vi "UHR-Fleezers Control (host) -Leonardo 04-2018 V3_greenctrl.vi"(0 "Tab Green FB":T5(tab)=enum."Trap Control (RF)") -> ()   [LabVIEW 2013] (continued)
                    n952 = call "Write to pump.vi"("string"="start", "VISA resource name"=w1530) -> ()  [unwired: 1 out]
                  }
                  frame #3 {
                    n953 = Wait (ms)(milliseconds to wait=u32 500) -> ()  [unwired: 1 out]
                  }
                  frame #4 {
                    n954 = call "Write to pump.vi"("string"="start", "VISA resource name"=w1534) -> ()  [unwired: 1 out]
                  }
                }
              }
            }
          }
          frame Enabled {
            n955 = call "hamilton_controller.vi"("Open?"=w1536, "valve"=enum16{"A", "B", "C", "D", "ALL"}."A", "action"=T21."MOVE VALVE") -> ()  [unwired: 8 in, 1 out]
          }
        }
      }
      event "Inject Valve B": Value Change {
        n956 = event-data() -> ()  [unwired: 7 out]
        n957 = disable-structure shown="Enabled" {
          disable-tunnel: "Inject Valve B" -> [w1540 w1560]
          frame Disabled {
            n958 = local read "Pump write delay (ms)"() -> (w1542:dbl)
            n959 = flat-sequence {
              tunnel: w1541 -> [w1555]
              tunnel: w1542 -> [w1551]
              tunnel: w1540 -> [_]
              tunnel: w1542 -> [w1557]
              tunnel: w1541 -> [w1558]
              frame #0 {
                n960 = local read "All Pump Parameters"() -> (w1550:T6)
                n961 = Multiply(x=60.0, y="Flush Center Ch Rate (ul/m)") -> (x*y=w1547:dbl)
                n962 = Unbundle By Name(w1550) -> ("Pump 2"=w1556:T33)
                n963 = call "Set pump parameters.vi"("Pump write delay (ms)"=w1551, "Volume (uL)"="Flush Center Ch Volume (uL)", "Rate (uL/h)"=w1547, "Units"=3.0, "Pump #"=2.0, "Pump Parameters In"=w1556, "VISA resource name"=w1555) -> ("Pump Parameters Out"=w1549:T33)  [unwired: 3 in]
                n964 = Bundle By Name(cluster=w1550, "Pump 2"=w1549) -> (w1548:T6)
                n965 = local write "All Pump Parameters"(w1548) -> ()
                n966 = Add(x="Flush Center Ch Volume (uL)", y="Total Volume\nFlushed (uL)") -> (x+y=w1544:dbl)
                n967 = local write "Total Volume\nFlushed (uL)"(w1544) -> ()
              }
              frame #1 {
                n968 = Wait (ms)(milliseconds to wait=w1557) -> ()  [unwired: 1 out]
              }
              frame #2 {
                n969 = call "Write to pump.vi"("string"="start", "VISA resource name"=w1558) -> ()  [unwired: 1 out]
              }
            }
            n970 = local read "Chemyx Syringe Pump Serial Port"() -> (w1541:refnum<visa-resource-name>)
          }
          frame Enabled {
            n971 = call "hamilton_controller.vi"("Open?"=w1560, "valve"=enum16{"A", "B", "C", "D", "ALL"}."B", "action"=T21."MOVE VALVE") -> ()  [unwired: 8 in, 1 out]
          }
        }
      }
      event "Inject Bottom": Value Change {
        n972 = event-data() -> ()  [unwired: 7 out]
        n973 = call "hamilton_controller.vi"("Open?"="Inject Bottom", "valve"=enum16{"A", "B", "C", "D", "ALL"}."C", "action"=T21."MOVE VALVE") -> ()  [unwired: 8 in, 1 out]
      }
      event "Shunt:": Value Change {
        n974 = event-data() -> ()  [unwired: 7 out]
        n975 = call "hamilton_controller.vi"("Open?"="Shunt:", "valve"=enum16{"A", "B", "C", "D", "ALL"}."D", "action"=T21."MOVE VALVE") -> ()  [unwired: 8 in, 1 out]
      }
      event "Flip Green Filter": Value Change {
        n976 = event-data() -> ()  [unwired: 7 out]
        n977 = local write "Flip Green Filter"("Flip Green Filter") -> ()
        n978 = flat-sequence {
          tunnel: w1576 -> [w1581]
          tunnel: w1575 -> [w1580]
          tunnel: [w1578] -> w1573
          tunnel: [w1577] -> w1572
          tunnel: [w1583] -> w1571
          tunnel: w1573 -> [w1583]
          tunnel: [w1582] -> w1570
          tunnel: w1572 -> [w1582]
          tunnel: w1571 -> [w1587]
          tunnel: w1570 -> [w1586]
          tunnel: [w1585] -> w1574
          frame #0 {
            n979 = xnode "Read/Write Control"("FPGA VI Reference In"=w1581, "error in"=w1580, "Green Filter Flipper"=TRUE) -> ("FPGA VI Reference Out"=w1578:T20, "error out"=w1577:errorcluster)
          }
          frame #1 {
            n980 = Wait (ms)(milliseconds to wait=u32 100) -> ()  [unwired: 1 out]
          }
          frame #2 {
            n981 = xnode "Read/Write Control"("FPGA VI Reference In"=w1587, "error in"=w1586, "Green Filter Flipper"=FALSE) -> ("error out"=w1585:errorcluster)  [unwired: 1 out]
          }
        }
      }
      event "Pump 1 contents", "Pump 3 contents": Value Change {
        n982 = event-data() -> ()  [unwired: 7 out]
        n983 = local read "Pump 1 contents"() -> (→"Pump 1 cont disp":string)
        n984 = local read "Pump 3 contents"() -> (→"Pump 3 cont disp":string)
      }
      event "Reset Trap Pos. FB": Value Change {
        n985 = event-data() -> ()  [unwired: 7 out]
        n986 = xnode "Read/Write Control"("FPGA VI Reference In"=w1593, "error in"=w1592, "Trap Pos. FB Reset"="Reset Trap Pos. FB") -> ()  [unwired: 2 out]
      }
      event "Trap Pos. FB ON": Value Change {
        n987 = event-data() -> ()  [unwired: 7 out]
        n988 = xnode "Read/Write Control"("FPGA VI Reference In"=w1608, "error in"=w1607) -> ("FPGA VI Reference Out"=w1605:T20, "BD1 Frequency Out 1"=w1602:u64)  [unwired: 1 out]
        n989 = To Double Precision Float(number=w1602) -> (double precision float=w1601:dbl)
        n990 = Multiply(x=49125000.0, y=6.0) -> (x*y=w1600:dbl)
        n991 = Multiply(x=w1601, y=w1600) -> (x*y=w1598:dbl)
        n992 = Scale By Power Of 2(n=-48, x=w1598) -> (x*2^n=w1597:dbl)
        n993 = Divide(x=w1597, y=1000000.0) -> (x/y=w1594:dbl)
        n994 = flat-sequence {
          tunnel: [w1611] -> w1606
          tunnel: w1605 -> [w1612]
          tunnel: w1602 -> [w1610]
          tunnel: "Trap Pos. FB ON" -> [w1609]
          tunnel: "Trap Pos. FB ON" -> [w1618]
          tunnel: w1606 -> [w1617]
          tunnel: "Trap Pos. FB ON" -> [w1620]
          tunnel: w1594 -> [w1619]
          frame #0 {
            n995 = case shown="False" w1609 {
              tunnel: w1612 -> [w1615 w1616]
              tunnel: [w1614 w1616] -> w1611
              tunnel: w1610 -> [w1613 _]
              frame False {
                n996 = xnode "Read/Write Control"("FPGA VI Reference In"=w1615, "BD 1 Frequency 1"=w1613) -> ("FPGA VI Reference Out"=w1614:T20)  [unwired: 1 in, 1 out]
              }
              frame True {
              }
            }
          }
          frame #1 {
            n997 = xnode "Read/Write Control"("FPGA VI Reference In"=w1617, "Force feedback"=w1618) -> ()  [unwired: 1 in, 2 out]
          }
          frame #2 {
            n998 = case shown="False" w1620 {
              tunnel: w1619 -> [w1623 _]
              frame False {
                n999 = local read "T2 for asymmetric\n(MHz)"() -> (w1621:dbl)
                n1000 = Subtract(x=w1621, y=w1623) -> (x-y=w1622:dbl)
                n1001 = property on="Trap Delta (MHz)" class="DigNum (strict)"("Val(Sgnl)"=w1622) -> ()  [unwired: 2 in, 2 out]
              }
              frame True {
              }
            }
          }
        }
      }
      event "Diff. FB.", "Trap Pos. FB Gains", "Trap Pos. FB Mult Factor", "Trap Pos. FB Offset Factor", "Trap Pos FB Negate Action", "Trap Pos FB Monitor\nT1 or T2", "Negate Diff?": Value Change {
        n1002 = event-data() -> ()  [unwired: 7 out]
        n1003 = xnode "Read/Write Control"("FPGA VI Reference In"=w1634, "error in"=w1633, "Trap pos. FB Range"="Trap Pos. FB Range", "Trap Pos. FB Gains"="Trap Pos. FB Gains", "Trap Pos. FB Mult Factor"="Trap Pos. FB Mult Factor", "Trap Pos. FB Offset Factor"="Trap Pos. FB Offset Factor", "Trap Pos FB Negate Action"="Trap Pos FB Negate Action", "Trap Pos FB Monitor T1 or T2"="Trap Pos FB Monitor\nT1 or T2", "AI1 X Scale"="Trap Pos. AI1 X Pre-scale", "Negate Diff?"="Negate Diff?", "Diff FB Measurement?"="Diff. FB.") -> ()  [unwired: 2 out]
      }
      event "Trap Pos FB SP": Value Change {
        n1004 = event-data() -> ()  [unwired: 7 out]
        n1005 = xnode "Read/Write Control"("FPGA VI Reference In"=w1637, "error in"=w1636, "Trap Pos. FB SP"="Trap Pos FB SP") -> ()  [unwired: 2 out]
        n1006 = disable-structure shown="Disabled" {
          frame Disabled {
            n1007 = local read "Trap X AI1 (DMA)"() -> (w1658:T13)
            n1008 = local read "Trap X (AI1)"() -> (w1659:T1)
            n1009 = local read "Setpoint offset\nCorrection values"() -> (w1652:dbl[])
            n1010 = local read "Trap Delta (MHz)"() -> (w1656:dbl)
            n1011 = local read "B factor"() -> (w1643:dbl)
            n1012 = Unbundle(w1659) -> ("Trap 1"=w1657:fxp<+/-,16,1>, "Trap 2"=w1646:fxp<+/-,16,1>)
            n1013 = Unbundle(w1658) -> ("Set 1"=w1642:fxp<+/-,16,1>, "Set 2"=w1641:fxp<+/-,16,1>)
            n1014 = Negate(x=w1646) -> (-x=w1639:fxp<+/-,17,2>)
            n1015 = Negate(x=w1657) -> (-x=w1640:fxp<+/-,17,2>)
            n1016 = Divide(x=w1656, y=0.1) -> (x/y=w1654:dbl)
            n1017 = Multiply(x=w1641, y=w1643) -> (x*y=w1644:dbl)
            n1018 = Subtract(x=w1642, y=w1644) -> (x-y=w1649:dbl)
            n1019 = To Long Integer(number=w1654) -> (32bit integer=w1653:i32)
            n1020 = Index Array(array=w1652, index=w1653) -> (element=w1648:dbl)
            n1021 = Multiply(x=w1643, y=w1639) -> (x*y=w1645:dbl)
            n1022 = Subtract(x=w1640, y=w1645) -> (x-y=w1651:dbl)
            n1023 = Add(x=w1651, y=w1648) -> (x+y=→"ideal setpoint fpga":dbl)
            n1024 = Add(x=w1649, y=w1648) -> (x+y=→"ideal setpoint avgd":dbl)
          }
          frame Enabled {
          }
        }
        n1025 = disable-structure shown="Enabled" {
          frame Enabled {
          }
          frame Disabled {
            n1026 = local write "B factor"(1.0 ("B factor")) -> ()
          }
        }
      }
      event "Simulate stepping": Value Change {
        n1027 = event-data() -> ()  [unwired: 7 out]
        n1028 = flat-sequence {
          tunnel: w1661 -> [w1664]
          tunnel: [w1663] -> _
          tunnel: w1660 -> [w1662]
          frame #0 {
            n1029 = while {
              tunnel: w1664 -> [w1692]
              tunnel: [w1691] -> w1663 mode=indexing
              tunnel: w1662 -> [w1690]
              i -> [w1676]
              stop <- w1673 stop-if-true
              w1666 = 1000.0
              n1030 = Divide(x="Backtrack probability", y=100) -> (x/y=w1700:dbl)
              n1031 = Random Number (0-1)() -> (number: 0 to 1=w1701:dbl)
              n1032 = Greater?(x=w1701, y=w1700) -> (0:w1699:bool)
              n1033 = Select(t=1, s=w1699, f=-1) -> (s? t:f=w1696:i32)
              n1034 = local read "BD 1 Frequency 2 (MHz)"() -> (w1671:dbl)
              n1035 = Multiply(x=w1696, y="Step size (nm)") -> (x*y=w1694:dbl)
              "Step taken" <- w1694
              n1036 = Divide(x=w1694, y=168.33) -> (x/y=w1669:dbl)
              n1037 = local read "BD 1 Frequency 1 (MHz)"() -> (w1670:dbl)
              n1038 = local read "X RF Frequency Limits (MHz)"() -> (w1689:T16)
              n1039 = local read "Y RF Frequency Limits (MHz)"() -> (w1688:T16)
              n1040 = Subtract(x=w1670, y=w1669) -> (x-y=w1668:dbl)
              n1041 = local write "BD 1 Frequency 1 (MHz)"(w1668) -> ()
              n1042 = local read "BD 2 Frequency 1 (MHz)"() -> (w1686:dbl)
              n1043 = local read "BD 2 Frequency 2 (MHz)"() -> (w1687:dbl)
              n1044 = call "set RF board frequency - interlace.vi"("Board 2 Frequency Limits"=w1688, "Board 1 Frequency Limits"=w1689, "error in"=w1692, "FPGA VI Reference In"=w1690, "Board 2 Frequency 2 (MHz)"=w1687, "Board 2 Frequency 1 (MHz)"=w1686, "Board 1 Frequency 2 (MHz)"=w1671, "Board 1 Frequency 1  (MHz)"=w1668) -> ("error out"=w1691:errorcluster)  [unwired: 2 in, 1 out]
              n1045 = Subtract(x=w1671, y=w1668) -> (x-y=w1685:dbl)
              n1046 = Subtract(x=w1687, y=w1686) -> (x-y=w1684:dbl)
              n1047 = Square(x=w1684) -> (x^2=w1682:dbl)
              n1048 = Square(x=w1685) -> (x^2=w1683:dbl)
              n1049 = Add(x=w1683, y=w1682) -> (x+y=w1681:dbl)
              n1050 = Square Root(x=w1681) -> (sqrt(x)=w1672:dbl)
              n1051 = local write "Trap Delta (MHz)"(w1672) -> ()
              n1052 = property on="Initial delta (MHz)" class="DigNum (strict)"("Val(Sgnl)"=w1672) -> ()  [unwired: 2 in, 2 out]
              n1053 = Multiply(x="Mean dwell time (s)", y=w1666) -> (x*y=w1678:dbl)
              n1054 = case shown="\"Gamma2\"" "Distribution" {
                tunnel: w1678 -> [w1705 w1709 w1712]
                tunnel: [w1705 w1706 w1713] -> w1667
                frame "uniform", Default {
                }
                frame "Exponential" {
                  n1055 = call-poly <vilib>:"Continuous Random.vi"("b"=w1709, "samples"=1) -> ("exp random data"=w1707:dbl[])  [unwired: 8 in, 1 out]
                  n1056 = Index Array(array=w1707) -> (element=w1706:dbl)  [unwired: 1 in]
                }
                frame "Gamma2" {
                  w1710 = 2.0
                  # "Note: the shape and scale\nparameters of the gamma\nare inverted because LabView..."
                  n1057 = Divide(x=w1712, y=w1710) -> (x/y=w1711:dbl)
                  n1058 = call-poly <vilib>:"Continuous Random.vi"("c"=w1711, "b"=w1710, "samples"=1) -> ("gamma random numbers"=w1714:dbl[])  [unwired: 7 in, 1 out]
                  n1059 = Index Array(array=w1714) -> (element=w1713:dbl)  [unwired: 1 in]
                }
              }
              n1060 = Divide(x=w1667, y=w1666) -> (x/y=→"Step duration":dbl)
              n1061 = To Unsigned Long Integer(number=w1667) -> (unsigned 32bit integer=w1679:u32)
              n1062 = Add(x=w1676, y=1) -> (x+y=w1675:i32)
              n1063 = Wait (ms)(milliseconds to wait=w1679) -> ()  [unwired: 1 out]
              n1064 = Equal?(x=w1675, y="Number of steps") -> (x = y?=w1673:bool)
            }
          }
          frame #1 {
            n1065 = local write "Simulate stepping"(FALSE) -> ()
          }
        }
      }
      event "Set SP to Reading": Value Change {
        n1066 = event-data() -> ()  [unwired: 7 out]
        n1067 = local read "Trap Pos FB Monitor\nT1 or T2"() -> (w1724:bool)
        n1068 = local read "Trap X AI1 (DMA)"() -> (w1727:T13)
        n1069 = local read "Trap X (AI1)"() -> (w1730:T1)
        n1070 = Unbundle By Name(w1730) -> ("Trap 1"=w1729:fxp<+/-,16,1>, "Trap 2"=w1728:fxp<+/-,16,1>)
        n1071 = Unbundle By Name(w1727) -> ("Set 1"=w1726:fxp<+/-,16,1>, "Set 2"=w1725:fxp<+/-,16,1>)
        n1072 = Select(t=w1729, s=w1724, f=w1728) -> (s? t:f=w1723:fxp<+/-,16,1>)
        n1073 = Select(t=w1726, s=w1724, f=w1725) -> (s? t:f=w1722:fxp<+/-,16,1>)
        n1074 = Not(x="Set SP Using...") -> (.not. x?=w1717:bool)
        n1075 = Select(t=w1723, s=w1717, f=w1722) -> (s? t:f=w1718:fxp<+/-,16,1>)
        n1076 = xnode "Read/Write Control"("FPGA VI Reference In"=w1720, "error in"=w1719, "Trap Pos. FB SP"=w1718) -> ()  [unwired: 2 out]
        n1077 = local write "Trap Pos FB SP"(w1718) -> ()
      }
      event "Trap Pos. FB Out Scale 2^n": Value Change {
        n1078 = event-data() -> ()  [unwired: 7 out]
        n1079 = Scale By Power Of 2(n="Trap Pos. FB Out Scale 2^n", x=ext 1.0) -> (x*2^n=w1732:ext)
        n1080 = property on="Trap Pos. FB Mult Factor" class="DigNum (strict)"("Val(Sgnl)"=w1732) -> ()  [unwired: 2 in, 2 out]
      }
      event "Trap Pos FB Int Count": Value Change {
        n1081 = event-data() -> ()  [unwired: 7 out]
        n1082 = xnode "Read/Write Control"("FPGA VI Reference In"=w1737, "error in"=w1736, "Trap Pos FB Int Count"="Trap Pos FB Int Count") -> ()  [unwired: 2 out]
      }
      event "Target Force (pN)", "Setpoint offset\nCorrection values", "Raster target force (pN)": Value Change {
        w1746 = 2.0
        n1083 = event-data() -> ()  [unwired: 7 out]
        n1084 = disable-structure "Removed B Factor to improve position feedback - Alex 081418 1of3" shown="Enabled" {
          disable-tunnel: [w1776 fxp<+/-,32,16> 1.0 ("B factor")] -> w1738
          frame Disabled {
            n1085 = local read "B factor"() -> (w1777:dbl)
            n1086 = To Fixed-Point(number=w1777) -> (fixed-point=w1776:fxp<+/-,16,16>)  [unwired: 1 in]
          }
          frame Enabled {
          }
        }
        n1087 = xnode "Read/Write Control"("FPGA VI Reference In"=w1740, "B factor"=w1738) -> ("BD1 Frequency Out 1"=w1767:u64)  [unwired: 1 in, 2 out]
        n1088 = local read "BD 1 Frequency 2 (MHz)"() -> (w1766:dbl)
        n1089 = local read "Target Force (pN)"() -> (w1752:dbl)
        n1090 = To Double Precision Float(number=w1767) -> (double precision float=w1773:dbl)
        n1091 = Multiply(x=49125000.0, y=6.0) -> (x*y=w1772:dbl)
        n1092 = Multiply(x=w1773, y=w1772) -> (x*y=w1770:dbl)
        n1093 = Scale By Power Of 2(n=-48, x=w1770) -> (x*2^n=w1769:dbl)
        n1094 = Divide(x=w1769, y=1000000.0) -> (x/y=w1765:dbl)
        n1095 = Subtract(x=w1766, y=w1765) -> (x-y=w1764:dbl)
        n1096 = local read "T1 kappa_x (pN/nm)"() -> (w1753:dbl)
        n1097 = local read "T1 alpha_x (nm/V)"() -> (w1754:dbl)
        n1098 = local read "Negate offset difference"() -> (w1755:bool)
        n1099 = local read "Offset file step size"() -> (w1763:dbl)
        n1100 = Multiply(x="Raster target force (pN)", y=w1746) -> (x*y=w1745:dbl)
        n1101 = Multiply(x=w1752, y=w1746) -> (x*y=w1751:dbl)
        n1102 = local read "Setpoint offset\nCorrection values"() -> (w1760:dbl[])
        n1103 = Divide(x=w1764, y=w1763) -> (x/y=w1762:dbl)
        n1104 = Select(t=-1, s=w1755, f=1) -> (s? t:f=w1756:i32)
        n1105 = To Long Integer(number=w1762) -> (32bit integer=w1761:i32)
        n1106 = Multiply(x=w1754, y=w1753) -> (x*y=w1744:dbl)
        n1107 = Divide(x=w1751, y=w1744) -> (x/y=w1750:dbl)
        n1108 = Index Array(array=w1760, index=w1761) -> (element=w1759:dbl)
        n1109 = Divide(x=w1745, y=w1744) -> (x/y=w1743:dbl)
        n1110 = Multiply(x=w1756, y=w1759) -> (x*y=w1742:dbl)
        n1111 = Add(x=w1750, y=w1742) -> (x+y=w1749:dbl)
        n1112 = Add(x=w1743, y=w1742) -> (x+y=w1741:dbl)
        n1113 = To Fixed-Point(number=w1741) -> (fixed-point=w1739:fxp<+/-,16,1>)  [unwired: 1 in]
        n1114 = To Fixed-Point(number=w1749) -> (fixed-point=w1748:fxp<+/-,16,1>)  [unwired: 1 in]
        n1115 = property on="Trap Pos FB SP" class="DigNum (strict)"("Val(Sgnl)"=w1748) -> ()  [unwired: 2 in, 2 out]
        n1116 = xnode "Read/Write Control"("FPGA VI Reference In"=w1740, "Raster setpoint"=w1739) -> ()  [unwired: 1 in, 2 out]
      }
      event "Read setpoint correction\nfile": Value Change {
        n1117 = event-data() -> ()  [unwired: 7 out]
        n1118 = local write "Read setpoint correction\nfile"(FALSE) -> ()
        n1119 = Open/Create/Replace File(file path (use dialog)="Setpoint correction\noffset file", operation (0:open)=T24."open", access (0:read/write)=enum16{"read/write", "read-only", "write-only"}."read-only") -> (refnum out=w1804:refnum<file>)  [unwired: 1 in, 4 out]
        n1120 = Deny Access(7:w1804) -> (3:w1802:refnum<file>)  [unwired: 1 in, 2 out]
        n1121 = Read from Binary File(5:0.0, 9:T30."big-endian, network order" ("byte order (0:big-endian, network order)"), 10:-1 ("count (1)"), 11:w1802) -> (2:w1795:dbl[], 3:w1801:refnum<file>)  [unwired: 1 in, 3 out]
        n1122 = Close File(refnum=w1801) -> ()  [unwired: 1 in, 2 out]
        n1123 = Index Array(array=w1795, index=0) -> (element=w1791:dbl)
        n1124 = local write "Offset file step size"(w1791) -> ()
        n1125 = Array Subset(array=w1795, index=3) -> (w1794:dbl[])  [unwired: 1 in]
        n1126 = local read "T1 kappa_x (pN/nm)"() -> (w1789:dbl)
        n1127 = local read "T1 alpha_x (nm/V)"() -> (w1790:dbl)
        n1128 = local read "T2 alpha_x (nm/V)"() -> (w1788:dbl)
        n1129 = local read "T2 kappa_x (pN/nm)"() -> (w1787:dbl)
        n1130 = Decimate 1D Array(w1794) -> (w1783:dbl[], w1784:dbl[])  [unwired: 1 out]
        n1131 = local read "Offset Values"() -> (w1793:T14)
        n1132 = Multiply(x=w1790, y=w1789) -> (x*y=w1785:dbl)
        n1133 = Multiply(x=w1788, y=w1787) -> (x*y=w1786:dbl)
        n1134 = Bundle By Name(cluster=w1793, "Trap 1X offset"=w1783, "Trap 2X offset"=w1784) -> (w1792:T14)
        n1135 = Divide(x=w1786, y=w1785) -> (x/y=w1780:dbl)
        n1136 = disable-structure "Removed B Factor to better position FB - Alex 081418 3of3" shown="Enabled" {
          disable-tunnel: w1780 -> [w1808 _]
          disable-tunnel: [w1808 1.0] -> w1779
          frame Disabled {
          }
          frame Enabled {
          }
        }
        n1137 = Multiply(x=w1784, y=w1779) -> (x*y=w1782:dbl[])
        n1138 = local write "Offset Values"(w1792) -> ()
        n1139 = Subtract(x=w1783, y=w1782) -> (x-y=w1781:dbl[])
        n1140 = property on="B factor" class="DigNum (strict)"("Val(Sgnl)"=w1779) -> ()  [unwired: 2 in, 2 out]
        n1141 = property on="Setpoint offset\nCorrection values" class="Arr (strict)"("Val(Sgnl)"=w1781) -> ()  [unwired: 2 in, 2 out]
      }
      event "MCL Tracking": Value Change {
        n1142 = event-data() -> ()  [unwired: 7 out]
        n1143 = case shown="True" "MCL Tracking" {
          frame False {
            n1144 = local read "Current MCL (V)"() -> (w1811:dbl)
            n1145 = local write "AO2"(w1811) -> ()
          }
          frame True {
            n1146 = local read "BD 1 Frequency 1 (MHz)"() -> (→"Zero T1 position":dbl)
            n1147 = local read "AO2"() -> (→"Zero MCL x position":dbl)
          }
        }
      }
      event "Scale intensities": Value Change {
        n1148 = event-data() -> ()  [unwired: 7 out]
        n1149 = local read "Trap Intensity\nSetpoints (V)"() -> (w1817:cluster{"Set 1":dbl, "Set 2":dbl})
        n1150 = local read "T1 kappa_x (pN/nm)"() -> (w1823:dbl)
        n1151 = local read "T2 kappa_x (pN/nm)"() -> (w1822:dbl)
        n1152 = Unbundle By Name(w1817) -> ("Set 1"=w1819:dbl, "Set 2"=w1818:dbl)
        n1153 = case shown="True" "Scale intensities" {
          tunnel: "Scale factor" -> [w1833 w1845]
          tunnel: "Scale factor" -> [w1828 w1838]
          tunnel: w1823 -> [w1835 w1844]
          tunnel: w1822 -> [w1834 w1843]
          tunnel: [w1831 w1842] -> w1821
          tunnel: [w1832 w1841] -> w1820
          tunnel: w1819 -> [w1830 w1840]
          tunnel: w1818 -> [w1829 w1839]
          tunnel: [w1827 w1837] -> w1816
          tunnel: [w1826 w1836] -> w1815
          frame False {
            n1154 = Divide(x=w1835, y=w1828) -> (x/y=w1831:dbl)
            n1155 = Divide(x=w1834, y=w1833) -> (x/y=w1832:dbl)
            n1156 = Divide(x=w1830, y=w1828) -> (x/y=w1827:dbl)
            n1157 = Divide(x=w1829, y=w1828) -> (x/y=w1826:dbl)
          }
          frame True {
            n1158 = Multiply(x=w1840, y=w1838) -> (x*y=w1837:dbl)
            n1159 = Multiply(x=w1839, y=w1838) -> (x*y=w1836:dbl)
            n1160 = Multiply(x=w1844, y=w1838) -> (x*y=w1842:dbl)
            n1161 = Multiply(x=w1845, y=w1843) -> (x*y=w1841:dbl)
          }
        }
        n1162 = local write "T2 kappa_x (pN/nm)"(w1820) -> ()
        n1163 = local write "T1 kappa_x (pN/nm)"(w1821) -> ()
        n1164 = Bundle By Name(cluster=w1817, "Set 1"=w1816, "Set 2"=w1815) -> (w1814:cluster{"Set 1":dbl, "Set 2":dbl})
        n1165 = property on="Trap Intensity\nSetpoints (V)" class="Clust (strict)"("Val(Sgnl)"=w1814) -> ()  [unwired: 2 in, 2 out]
      }
    }
    "error out 2" <- w772
    n1166 = node-c288() -> ()  [unwired: 1 in, 1 out]
  }
  n1167 = node-c288() -> (w103:T25)  [unwired: 4 in]
  n1168 = timed-loop "Run Scripts, including: stage motion" {
    timing: w103 -> [_]
    timing-out: [_] -> w102
    tunnel: w61 -> [_]
    stop <- w1847 stop-if-true
    n1169 = node-c288() -> ()  [unwired: 1 in, 1 out]
    n1170 = event shown="[0] \"Move Cap. 1 (DNA Top)\": Value Change" {
      selector: _ -> [_ _ _ _ _ _ _ _ _ _ _ _]
      dyn-events: _ -> [_ _ _ _ _ _ _ _ _ _ _ _]
      timeout: 50 -> [_ _ _ _ _ _ _ _ _ _ _ _]
      tunnel: ["Move Cap. 1 (DNA Top)" _ "Cal/Data Acq. Spot" "Dump Beads" "Dip for Protein" _ "Got ADig bead" "Got DNA bead" "Take Stepping Data" _ "Take Detection Laser\nImage" _] -> _
      tunnel: [_ _ _ _ _ _ _ _ _ _ _ w2057] -> w1847
      event "Move Cap. 1 (DNA Top)": Value Change {
        n1171 = event-data() -> ()  [unwired: 1 in, 5 out]
        n1172 = local write "Move Cap. 1 (DNA Top)"(FALSE ("Move Cap. 1 (DNA Right)")) -> ()
        n1173 = flat-sequence {
          tunnel: "Cap 1 Samp Flow ON" -> [w1853]
          frame #0 {
            n1174 = local write "Stage Moving"(FALSE ("Stage Moving")) -> ()
            n1175 = case "stop flow" shown="True" w1853 {
              frame False {
              }
              frame True {
                n1176 = call "hamilton_controller.vi"("Open?"=FALSE, "valve"=enum16{"A", "B", "C", "D", "ALL"}."C", "action"=T21."MOVE VALVE") -> ()  [unwired: 8 in, 1 out]
              }
            }
            n1177 = case shown="True" TRUE {
              tunnel: "Cap 1 T ON" -> [w1862 w1863]
              frame False {
                n1178 = property on="Trap 1 (ON/OFF)" class="Bool (strict)"("Val(Sgnl)"=w1862) -> ()  [unwired: 2 in, 2 out]
              }
              frame True {
                n1179 = property on="Trap 2 (ON/OFF)" class="Bool (strict)"("Val(Sgnl)"=w1863) -> ()  [unwired: 2 in, 2 out]
              }
            }
            n1180 = call <vilib>:"Beep.vi"() -> ()  [unwired: 3 in, 9 out]
            n1181 = case shown="True" "Cap 1 Flow ON" {
              frame False {
              }
              frame True {
                n1182 = property on="Main:" class="Bool (strict)"("Val(Sgnl)"=TRUE ("Value (Signaling)")) -> ()  [unwired: 2 in, 2 out]
              }
            }
          }
        }
      }
      event Timeout {
        n1183 = event-data() -> ()  [unwired: 1 in, 2 out]
      }
      event "Cal/Data Acq. Spot": Value Change {
        # "wait for calibration file\nto be written"
        # "signal save cal true\nthis tells the data \nacquisition loop to\nstart sending the data\nto a calibration file"
        # "separate traps to\nthe desired trap delta"
        # "move stage to data acquisition spot"
        # "CHANGE FISH FOR TETHER BACK\nTO TRUE VALUE HERE."
        n1184 = event-data() -> ()  [unwired: 1 in, 5 out]
        n1185 = flat-sequence {
          tunnel: ["Cal @ (MHz)"] -> w1864
          tunnel: w1864 -> [w1876]
          tunnel: w1864 -> [w1897]
          frame #0 {
            n1186 = property on="Trap Delta (MHz)" class="DigNum (strict)"("Val(Sgnl)"="Cal @ (MHz)") -> ()  [unwired: 2 in, 2 out]
            n1187 = call <vilib>:"Beep.vi"() -> ()  [unwired: 3 in, 9 out]
          }
          frame #1 {
            n1188 = local read "Scale intensities"() -> (w1868:bool)
            n1189 = case shown="True" w1868 {
              frame False {
              }
              frame True {
                n1190 = property on="Scale intensities" class="Bool (strict)"("Val(Sgnl)"=FALSE ("Value (Signaling)")) -> ()  [unwired: 2 in, 2 out]
              }
            }
          }
          frame #2 {
            n1191 = Wait (ms)(milliseconds to wait=u32 500) -> ()  [unwired: 1 out]
          }
          frame #3 {
            n1192 = property on="Save Calibration" class="Bool (strict)"("Val(Sgnl)"=TRUE ("Value (Signaling)")) -> ()  [unwired: 2 in, 2 out]
          }
          frame #4 {
            n1193 = Wait (ms)(milliseconds to wait=u32 4000) -> ()  [unwired: 1 out]
          }
          frame #5 {
            n1194 = while {
              stop <- w1873 stop-if-true
              n1195 = local read "Saving..."() -> (w1874:bool)
              n1196 = Wait (ms)(milliseconds to wait=u32 100) -> ()  [unwired: 1 out]
              n1197 = Not(x=w1874) -> (.not. x?=w1873:bool)
            }
          }
          frame #6 {
            n1198 = case shown="True" "W/ Offset 1" {
              tunnel: w1876 -> [_ w1878]
              frame False {
              }
              frame True {
                n1199 = stacked-sequence {
                  tunnel: w1878 -> [_ _ _ _ _ _ _ w1895]
                  frame #0 {
                    n1200 = Replace Array Subset(array=u32[] [0] ("Index Values"), new element="Offset 1 Set", index=0) -> (w1879:u32[])
                    n1201 = property on="Saved AOD Raster Scan Parameter Sets" class="Arr (strict)"("Index Values"=w1879) -> ()  [unwired: 2 in, 2 out]
                    n1202 = property on="Trap Delta (MHz)" class="DigNum (strict)"("Val(Sgnl)"="Offset 1 Start (MHz)") -> ()  [unwired: 2 in, 2 out]
                  }
                  frame #1 {
                    n1203 = Wait (ms)(milliseconds to wait=u32 200) -> ()  [unwired: 1 out]
                  }
                  frame #2 {
                    n1204 = property on="Load parameters" class="Bool (strict)"("Val(Sgnl)"=TRUE ("Value (Signaling)")) -> ()  [unwired: 2 in, 2 out]
                  }
                  frame #3 {
                    n1205 = Wait (ms)(milliseconds to wait=u32 200) -> ()  [unwired: 1 out]
                  }
                  frame #4 {
                    n1206 = property on="Trap Raster Scan" class="Bool (strict)"("Val(Sgnl)"=TRUE ("Value (Signaling)")) -> ()  [unwired: 2 in, 2 out]
                  }
                  frame #5 {
                    n1207 = Wait (ms)(milliseconds to wait=u32 2000) -> ()  [unwired: 1 out]
                  }
                  frame #6 {
                    n1208 = while {
                      stop <- w1892 stop-if-true
                      n1209 = local read "Raster Scanning..."() -> (w1894:bool)
                      n1210 = local read "Saving..."() -> (w1890:bool)
                      n1211 = Wait (ms)(milliseconds to wait=u32 100) -> ()  [unwired: 1 out]
                      n1212 = Not(x=w1890) -> (.not. x?=w1889:bool)
                      n1213 = Not(x=w1894) -> (.not. x?=w1891:bool)
                      n1214 = And(x=w1891, y=w1889) -> (x .and. y?=w1892:bool)
                    }
                  }
                  frame #7 {
                    n1215 = property on="Trap Delta (MHz)" class="DigNum (strict)"("Val(Sgnl)"=w1895) -> ()  [unwired: 2 in, 2 out]
                  }
                }
              }
            }
          }
          frame #7 {
            n1216 = local read "Save ave N"() -> (w1896:dbl)
            n1217 = case shown="True" "W/ Offset 2" {
              tunnel: w1897 -> [_ w1903]
              tunnel: w1896 -> [_ w1902]
              frame False {
                n1218 = Multiply(x="Cal read wait (s)", y=u32 1000 ("milliseconds to wait")) -> (x*y=w1900:u32)
                n1219 = Wait (ms)(milliseconds to wait=w1900) -> ()  [unwired: 1 out]
              }
              frame True {
                n1220 = stacked-sequence {
                  tunnel: w1903 -> [_ _ _ _ _ _ _ _ _ w1924 _ _]
                  tunnel: w1902 -> [_ _ _ _ _ _ _ _ _ w1922 _ _]
                  frame #0 {
                    n1221 = property on="Save ave N" class="DigNum (strict)"("Val(Sgnl)"=1.0 ("Value (Signaling)")) -> ()  [unwired: 2 in, 2 out]
                  }
                  frame #1 {
                    n1222 = Wait (ms)(milliseconds to wait=u32 500) -> ()  [unwired: 1 out]
                  }
                  frame #2 {
                    n1223 = property on="Trap Delta (MHz)" class="DigNum (strict)"("Val(Sgnl)"="Offset 2 Start (MHz)") -> ()  [unwired: 2 in, 2 out]
                    n1224 = Replace Array Subset(array=u32[] [0] ("Index Values"), new element="Offset 2 Set", index=0) -> (w1908:u32[])
                    n1225 = property on="Saved AOD Raster Scan Parameter Sets" class="Arr (strict)"("Index Values"=w1908) -> ()  [unwired: 2 in, 2 out]
                  }
                  frame #3 {
                    n1226 = Wait (ms)(milliseconds to wait=u32 500) -> ()  [unwired: 1 out]
                  }
                  frame #4 {
                    n1227 = property on="Load parameters" class="Bool (strict)"("Val(Sgnl)"=TRUE ("Value (Signaling)")) -> ()  [unwired: 2 in, 2 out]
                  }
                  frame #5 {
                    n1228 = Wait (ms)(milliseconds to wait=u32 500) -> ()  [unwired: 1 out]
                  }
                  frame #6 {
                    n1229 = property on="Trap Raster Scan" class="Bool (strict)"("Val(Sgnl)"=TRUE ("Value (Signaling)")) -> ()  [unwired: 2 in, 2 out]
                  }
                  frame #7 {
                    n1230 = Wait (ms)(milliseconds to wait=u32 2000) -> ()  [unwired: 1 out]
                  }
                  frame #8 {
                    n1231 = while {
                      stop <- w1917 stop-if-true
                      n1232 = local read "Raster Scanning..."() -> (w1920:bool)
                      n1233 = local read "Saving..."() -> (w1918:bool)
                      n1234 = Wait (ms)(milliseconds to wait=u32 100) -> ()  [unwired: 1 out]
                      n1235 = Not(x=w1918) -> (.not. x?=w1916:bool)
                      n1236 = Not(x=w1920) -> (.not. x?=w1919:bool)
                      n1237 = And(x=w1919, y=w1916) -> (x .and. y?=w1917:bool)
                    }
                  }
                  frame #9 {
                    n1238 = property on="Trap Delta (MHz)" class="DigNum (strict)"("Val(Sgnl)"=w1924) -> ()  [unwired: 2 in, 2 out]
                    n1239 = property on="Saved AOD Raster Scan Parameter Sets" class="Arr (strict)"("Index Values"=u32[] [0]) -> ()  [unwired: 2 in, 2 out]
                    n1240 = property on="Save ave N" class="DigNum (strict)"("Val(Sgnl)"=w1922) -> ()  [unwired: 2 in, 2 out]
                  }
                  frame #10 {
                    n1241 = Wait (ms)(milliseconds to wait=u32 500) -> ()  [unwired: 1 out]
                  }
                  frame #11 {
                    n1242 = property on="Load parameters" class="Bool (strict)"("Val(Sgnl)"=TRUE ("Value (Signaling)")) -> ()  [unwired: 2 in, 2 out]
                  }
                }
              }
            }
          }
          frame #8 {
            n1243 = property on="Read Cal" class="Bool (strict)"("Val(Sgnl)"=TRUE ("Value (Signaling)")) -> ()  [unwired: 2 in, 2 out]
          }
          frame #9 {
            n1244 = Wait (ms)(milliseconds to wait=u32 500) -> ()  [unwired: 1 out]
          }
          frame #10 {
            n1245 = property on="Fish for Tether" class="Bool (strict)"("Val(Sgnl)"=FALSE ("Value (Signaling)")) -> ()  [unwired: 2 in, 2 out]
          }
        }
        n1246 = local write "Cal/Data Acq. Spot"(FALSE ("Cal/Data Acq. Spot")) -> ()
      }
      event "Dump Beads": Value Change {
        # "SCRIPT TO REMOVE BOTH BEADS FROM THE TRAPS. TURNS ON LIGHT WHICH INDICATES THAT STAGE IS MOVING. THEN STOPS SAVING DATA. \nSETS Sample Channel Flow TO TRUE. STOPS INTERLACING GREEN FLUORESCENCE. TURNS OFF Tether INDICATOR BECAUSE WE ARE THROWING IT\nAWAY. SHUTS OFF TRAP POSITION FEEDBACK."
        n1247 = event-data() -> ()  [unwired: 1 in, 5 out]
        n1248 = flat-sequence {
          frame #0 {
            w1931 = FALSE ("Fl. Triggered...")
            w1932 = TRUE ("Stage Moving")
            n1249 = local read "Saving..."() -> (w1933:bool)
            n1250 = local write "Fl. Triggered..."(w1931) -> ()
            n1251 = local write "Stage Moving"(w1932) -> ()
            n1252 = local write "Tether"(w1931) -> ()
            n1253 = property on="Green Laser ON/Interlacing" class="Bool (strict)"("Val(Sgnl)"=w1931) -> ()  [unwired: 2 in, 2 out]
            n1254 = property on="Trap Pos. FB ON" class="Bool (strict)"("Val(Sgnl)"=w1931) -> ()  [unwired: 2 in, 2 out]
            n1255 = property on="Inject Bottom" class="Bool (strict)"("Val(Sgnl)"=w1932) -> ()  [unwired: 2 in, 2 out]
            n1256 = local write "Stop Saving"(w1933) -> ()
          }
          frame #1 {
            w1934 = FALSE ("Value (Signaling)")
            # "TURNS TRAPS OFF SO THAT\nBEADS REMAIN AT DUMP \nBEADS POSITION"
            n1257 = property on="Trap 1 (ON/OFF)" class="Bool (strict)"("Val(Sgnl)"=w1934) -> ()  [unwired: 2 in, 2 out]
            n1258 = property on="Trap 2 (ON/OFF)" class="Bool (strict)"("Val(Sgnl)"=w1934) -> ()  [unwired: 2 in, 2 out]
            n1259 = call <vilib>:"Beep.vi"() -> ()  [unwired: 3 in, 9 out]
          }
          frame #2 {
            n1260 = property on="Goto Bottom (F7)" class="Bool"("Val(Sgnl)"=TRUE ("Value (Signaling)")) -> ()  [unwired: 2 in, 2 out]
          }
          frame #3 {
            n1261 = Wait (ms)(milliseconds to wait=u32 8000) -> ()  [unwired: 1 out]
          }
          frame #4 {
            n1262 = property on="Trap Delta (MHz)" class="DigNum (strict)"("Val(Sgnl)"=20.0 ("Value (Signaling)")) -> ()  [unwired: 2 in, 2 out]
          }
          frame #5 {
            n1263 = property on="Trap 2 (ON/OFF)" class="Bool (strict)"("Val(Sgnl)"=TRUE ("Value (Signaling)")) -> ()  [unwired: 2 in, 2 out]
          }
          frame #6 {
            n1264 = property on="Inject Bottom" class="Bool (strict)"("Val(Sgnl)"=FALSE ("Value (Signaling)")) -> ()  [unwired: 2 in, 2 out]
          }
        }
      }
      event "Dip for Protein": Value Change {
        n1265 = event-data() -> ()  [unwired: 1 in, 5 out]
        n1266 = flat-sequence {
          frame #0 {
            n1267 = case shown="True" "Move Trap Before?" {
              frame False {
              }
              frame True {
                n1268 = property on="Trap Delta (MHz)" class="DigNum (strict)"("Val(Sgnl)"="Dip Trap Delta 1 (MHz)") -> ()  [unwired: 2 in, 2 out]
              }
            }
          }
          frame #1 {
            n1269 = Multiply(x="Duration (s)", y=1000.0) -> (x*y=w1943:dbl)
            n1270 = Wait (ms)(milliseconds to wait=w1943) -> ()  [unwired: 1 out]
          }
          frame #2 {
            n1271 = case shown="True" "Move Trap After?" {
              frame False {
              }
              frame True {
                n1272 = property on="Trap Delta (MHz)" class="DigNum (strict)"("Val(Sgnl)"="Dip Trap Delta 2 (MHz)") -> ()  [unwired: 2 in, 2 out]
              }
            }
          }
          frame #3 {
            n1273 = case shown="True" "Green ON After?" {
              frame False {
              }
              frame True {
                n1274 = property on="Green Laser ON/Interlacing" class="Bool (strict)"("Val(Sgnl)"=TRUE ("Value (Signaling)")) -> ()  [unwired: 2 in, 2 out]
              }
            }
          }
          frame #4 {
            n1275 = Wait (ms)(milliseconds to wait=u32 500) -> ()  [unwired: 1 out]
          }
          frame #5 {
            n1276 = case shown="True" "Save Data After?" {
              frame False {
              }
              frame True {
                n1277 = property on="Start Saving" class="Bool (strict)"("Val(Sgnl)"=TRUE ("Value (Signaling)")) -> ()  [unwired: 2 in, 2 out]
              }
            }
          }
        }
      }
      event "Profile": Value Change {
        n1278 = event-data() -> ()  [unwired: 1 in, 5 out]
        n1279 = flat-sequence {
          frame #0 {
            w1953 = 0.0 ("element")
            n1280 = Build Array(w1953, "Y change (mm)", w1953) -> ()  [unwired: 1 out]
          }
          frame #1 {
            # "stop saving"
            n1281 = local write "Stop Saving"(TRUE ("Stop Saving")) -> ()
            n1282 = local write "Stage Moving"(FALSE ("Stage Moving")) -> ()
          }
        }
      }
      event "Got ADig bead": Value Change {
        n1283 = event-data() -> ()  [unwired: 1 in, 5 out]
        n1284 = property on="Move Cap. 1 (DNA Top)" class="Bool (strict)"("Val(Sgnl)"=TRUE ("Value (Signaling)")) -> ()  [unwired: 2 in, 2 out]
        n1285 = property on="Inject Top:" class="Bool (strict)"("Val(Sgnl)"=FALSE ("Value (Signaling)")) -> ()  [unwired: 2 in, 2 out]
      }
      event "Got DNA bead": Value Change {
        n1286 = event-data() -> ()  [unwired: 1 in, 5 out]
        n1287 = property on="Cal/Data Acq. Spot" class="Bool (strict)"("Val(Sgnl)"=TRUE ("Value (Signaling)")) -> ()  [unwired: 2 in, 2 out]
        n1288 = property on="Main:" class="Bool (strict)"("Val(Sgnl)"=FALSE ("Value (Signaling)")) -> ()  [unwired: 2 in, 2 out]
      }
      event "Take Stepping Data": Value Change {
        n1289 = event-data() -> ()  [unwired: 1 in, 5 out]
        n1290 = local read "Save ave N"() -> (w1971:dbl)
        n1291 = flat-sequence {
          tunnel: w1971 -> [w1973]
          tunnel: [w1973] -> w1966
          tunnel: [w1975] -> w1967
          tunnel: w1966 -> [w1975]
          tunnel: [w1977] -> w1968
          tunnel: w1967 -> [w1977]
          tunnel: [w1980] -> w1969
          tunnel: w1968 -> [w1980]
          tunnel: [w1982] -> w1970
          tunnel: w1969 -> [w1982]
          tunnel: [w1984] -> w1964
          tunnel: w1970 -> [w1984]
          tunnel: w1964 -> [w1987]
          tunnel: [w1987] -> w1963
          tunnel: w1963 -> [w1988]
          tunnel: [w1988] -> w1965
          tunnel: w1965 -> [w1994]
          frame #0 {
            n1292 = property on="Save ave N" class="DigNum (strict)"("Val(Sgnl)"="Save ave factor") -> ()  [unwired: 2 in, 2 out]
          }
          frame #1 {
            n1293 = Wait (ms)(milliseconds to wait=u32 100) -> ()  [unwired: 1 out]
          }
          frame #2 {
            n1294 = local read "Offset 2 Start (MHz)"() -> (w1979:dbl)
            n1295 = property on="Saved AOD Raster Scan Parameter Sets" class="Arr (strict)"("Index Values"=u32[] [2]) -> ()  [unwired: 2 in, 2 out]
            n1296 = property on="Trap Delta (MHz)" class="DigNum (strict)"("Val(Sgnl)"=w1979) -> ()  [unwired: 2 in, 2 out]
          }
          frame #3 {
            n1297 = property on="Load parameters" class="Bool (strict)"("Val(Sgnl)"=TRUE ("Value (Signaling)")) -> ()  [unwired: 2 in, 2 out]
          }
          frame #4 {
            n1298 = Wait (ms)(milliseconds to wait=u32 100) -> ()  [unwired: 1 out]
          }
          frame #5 {
            n1299 = property on="Trap Raster Scan" class="Bool (strict)"("Val(Sgnl)"=TRUE ("Value (Signaling)")) -> ()  [unwired: 2 in, 2 out]
          }
          frame #6 {
            n1300 = Wait (ms)(milliseconds to wait=u32 1000) -> ()  [unwired: 1 out]
          }
          frame #7 {
            n1301 = while {
              stop <- w1991 stop-if-true
              n1302 = local read "Raster Scanning..."() -> (w1993:bool)
              n1303 = local read "Saving..."() -> (w1992:bool)
              n1304 = Not(x=w1992) -> (.not. x?=w1989:bool)
              n1305 = Not(x=w1993) -> (.not. x?=w1990:bool)
              n1306 = And(x=w1990, y=w1989) -> (x .and. y?=w1991:bool)
            }
          }
          frame #8 {
            n1307 = property on="Save ave N" class="DigNum (strict)"("Val(Sgnl)"=w1994) -> ()  [unwired: 2 in, 2 out]
          }
        }
      }
      event "Step Size (nm)": Value Change {
        n1308 = event-data() -> ()  [unwired: 1 in, 5 out]
        n1309 = flat-sequence {
          frame #0 {
            n1310 = property on="Saved AOD Raster Scan Parameter Sets" class="Arr (strict)"("Index Values"=u32[] [1]) -> ()  [unwired: 2 in, 2 out]
          }
          frame #1 {
            n1311 = Multiply(x="N Steps", y="Step Size (nm)") -> (x*y=w1996:dbl)
            n1312 = property on="Scan Speed AOD (nm/s) 2" class="DigNum (strict)"("Value"="Step Size (nm)") -> ()  [unwired: 2 in, 2 out]
            n1313 = property on="Step Size AOD (nm) 2" class="DigNum (strict)"("Value"="Step Size (nm)") -> ()  [unwired: 2 in, 2 out]
            n1314 = property on="Scan Range AOD (nm) 2" class="DigNum (strict)"("Value"=w1996) -> ()  [unwired: 2 in, 2 out]
          }
        }
      }
      event "Take Detection Laser\nImage": Value Change {
        n1315 = event-data() -> ()  [unwired: 1 in, 5 out]
        n1316 = flat-sequence {
          tunnel: [w2024] -> w2014
          tunnel: [w2023] -> w2007
          tunnel: [w2022] -> w1999
          tunnel: [w2027] -> w2015
          tunnel: w2014 -> [w2027]
          tunnel: [w2026] -> w2008
          tunnel: w2007 -> [w2026]
          tunnel: [w2025] -> w2000
          tunnel: w1999 -> [w2025]
          tunnel: [w2031] -> w2016
          tunnel: w2015 -> [w2031]
          tunnel: [w2030] -> w2009
          tunnel: w2008 -> [w2030]
          tunnel: [w2029] -> w2001
          tunnel: w2000 -> [w2029]
          tunnel: [w2037] -> w2017
          tunnel: w2016 -> [w2037]
          tunnel: [w2036] -> w2010
          tunnel: w2009 -> [w2036]
          tunnel: [w2035] -> w2002
          tunnel: w2001 -> [w2035]
          tunnel: [w2041] -> w2018
          tunnel: w2017 -> [w2041]
          tunnel: [w2040] -> w2011
          tunnel: w2010 -> [w2040]
          tunnel: [w2039] -> w2003
          tunnel: w2002 -> [w2039]
          tunnel: [w2045] -> w2019
          tunnel: w2018 -> [w2045]
          tunnel: [w2044] -> w2012
          tunnel: w2011 -> [w2044]
          tunnel: [w2043] -> w2004
          tunnel: w2003 -> [w2043]
          tunnel: [w2049] -> w2020
          tunnel: w2019 -> [w2049]
          tunnel: [w2048] -> w2013
          tunnel: w2012 -> [w2048]
          tunnel: [w2047] -> w2005
          tunnel: w2004 -> [w2047]
          tunnel: w2020 -> [w2055]
          tunnel: w2013 -> [w2054]
          tunnel: [w2052] -> w2006
          tunnel: w2005 -> [w2052]
          tunnel: w2006 -> [w2056]
          frame #0 {
            n1317 = local read "Green Laser ON/Interlacing"() -> (w2024:bool)
            n1318 = local read "Green laser mode"() -> (w2023:enum32{"Laser ON", "Laser OFF", "Interlace"})
            n1319 = local read "Green FB On/Off"() -> (w2022:bool)
          }
          frame #1 {
            n1320 = property on="Green FB On/Off" class="Bool (strict)"("Val(Sgnl)"=FALSE ("Value (Signaling)")) -> ()  [unwired: 2 in, 2 out]
          }
          frame #2 {
            n1321 = property on="Green Laser ON/Interlacing" class="Bool (strict)"("Val(Sgnl)"=TRUE ("Value (Signaling)")) -> ()  [unwired: 2 in, 2 out]
            n1322 = property on="Flip Green Filter" class="Bool (strict)"("Val(Sgnl)"=TRUE ("Value (Signaling)")) -> ()  [unwired: 2 in, 2 out]
            n1323 = property on="Green laser mode" class="RadioBtnsControl (strict)"("Val(Sgnl)"=enum32{"Laser ON", "Laser OFF", "Interlace"}."Laser ON" ("Value (Signaling)")) -> ()  [unwired: 2 in, 2 out]
          }
          frame #3 {
            n1324 = Wait (ms)(milliseconds to wait=u32 500) -> ()  [unwired: 1 out]
          }
          frame #4 {
            n1325 = property on="Confocal Image" class="Bool (strict)"("Val(Sgnl)"=TRUE ("Value (Signaling)")) -> ()  [unwired: 2 in, 2 out]
          }
          frame #5 {
            n1326 = Wait (ms)(milliseconds to wait=u32 2000) -> ()  [unwired: 1 out]
          }
          frame #6 {
            n1327 = while {
              stop <- w2050 stop-if-true
              n1328 = local read "Saving..."() -> (w2051:bool)
              n1329 = Not(x=w2051) -> (.not. x?=w2050:bool)
            }
          }
          frame #7 {
            n1330 = property on="Flip Green Filter" class="Bool (strict)"("Val(Sgnl)"=TRUE ("Value (Signaling)")) -> ()  [unwired: 2 in, 2 out]
            n1331 = property on="Green Laser ON/Interlacing" class="Bool (strict)"("Val(Sgnl)"=w2055) -> ()  [unwired: 2 in, 2 out]
            n1332 = property on="Green laser mode" class="RadioBtnsControl (strict)"("Val(Sgnl)"=w2054) -> ()  [unwired: 2 in, 2 out]
          }
          frame #8 {
            n1333 = property on="Green FB On/Off" class="Bool (strict)"("Val(Sgnl)"=w2056) -> ()  [unwired: 2 in, 2 out]
          }
        }
      }
      event "Stop All": Value Change {
        n1334 = event-data() -> ()  [unwired: 1 in, 5 out]
        n1335 = local read "Stop All"() -> (w2057:bool)
      }
    }
    n1336 = node-c288() -> ()  [unwired: 1 in, 1 out]
  }
  n1337 = node-c288() -> (w110:T25)  [unwired: 4 out]
  n1338 = timed-loop "Mouse control: trap position (AOM deflection), set confocal spot from image" {
    tunnel: [w2059] -> w70
    tunnel: w61 -> [w2058]
    timing: w110 -> [_]
    timing-out: [_] -> w109
    stop <- w2059 stop-if-true
    n1339 = node-c288() -> ()  [unwired: 2 out]
    n1340 = event shown="[0] \"Pane\": Mouse Down" {
      selector: _ -> [_ _]
      dyn-events: _ -> [_ _]
      timeout: _ -> [_ _]
      tunnel: w2058 -> [w2062 _]
      event Mouse Down {
        n1341 = event-data() -> ("Time"=w2064:u32, "Coords"=w2063:T8, "Button"=w2065:u16)  [unwired: 6 out]
        n1342 = case shown="1" w2065 {
          tunnel: w2064 -> [_ _ w2168]
          tunnel: w2063 -> [_ w2102 w2166]
          tunnel: w2062 -> [_ _ w2164]
          frame 0, Default {
          }
          frame 1 {
            n1343 = property on="APD 2" class="ImageControl"() -> ("Displayed Image Position"=w2072:cluster{"Left":i32, "Top":i32})  [unwired: 2 in, 2 out]
            n1344 = property on="APD 1" class="ImageControl"() -> ("Displayed Image Position"=w2101:cluster{"Left":i32, "Top":i32})  [unwired: 2 in, 2 out]
            n1345 = property on="Detection Laser X" class="ImageControl"() -> ("Displayed Image Position"=w2098:cluster{"Left":i32, "Top":i32})  [unwired: 2 in, 2 out]
            n1346 = property on="Detection Laser Y" class="ImageControl"() -> ("Displayed Image Position"=w2097:cluster{"Left":i32, "Top":i32})  [unwired: 2 in, 2 out]
            n1347 = property on="APD 2" class="ImageControl"() -> ("Displayed Image Size"=w2071:cluster{"Width":u32, "Height":u32})  [unwired: 2 in, 2 out]
            n1348 = property on="APD 1" class="ImageControl"() -> ("Displayed Image Size"=w2099:cluster{"Width":u32, "Height":u32})  [unwired: 2 in, 2 out]
            n1349 = property on="Detection Laser X" class="ImageControl"() -> ("Displayed Image Size"=w2100:cluster{"Width":u32, "Height":u32})  [unwired: 2 in, 2 out]
            n1350 = property on="Detection Laser Y" class="ImageControl"() -> ("Displayed Image Size"=w2096:cluster{"Width":u32, "Height":u32})  [unwired: 2 in, 2 out]
            n1351 = Unbundle By Name(w2071) -> ("Width"=w2068:u32, "Height"=w2067:u32)
            n1352 = Unbundle By Name(w2072) -> ("Left"=w2070:i32, "Top"=w2069:i32)
            n1353 = Unbundle By Name(w2099) -> ("Width"=w2093:u32, "Height"=w2092:u32)
            n1354 = Unbundle By Name(w2100) -> ("Width"=w2089:u32, "Height"=w2088:u32)
            n1355 = Unbundle By Name(w2096) -> ("Width"=w2085:u32, "Height"=w2084:u32)
            n1356 = Unbundle By Name(w2101) -> ("Left"=w2095:i32, "Top"=w2094:i32)
            n1357 = Unbundle By Name(w2098) -> ("Left"=w2091:i32, "Top"=w2090:i32)
            n1358 = Unbundle By Name(w2097) -> ("Left"=w2087:i32, "Top"=w2086:i32)
            n1359 = Bundle("Left"=w2070, "Top"=w2069, "Width"=w2068, "Height"=w2067) -> (w2066:T34)  [unwired: 1 in]
            n1360 = Bundle("Left"=w2095, "Top"=w2094, "Width"=w2093, "Height"=w2092) -> (w2083:T34)  [unwired: 1 in]
            n1361 = Bundle("Left"=w2091, "Top"=w2090, "Width"=w2089, "Height"=w2088) -> (w2082:T34)  [unwired: 1 in]
            n1362 = Bundle("Left"=w2087, "Top"=w2086, "Width"=w2085, "Height"=w2084) -> (w2081:T34)  [unwired: 1 in]
            n1363 = Build Cluster Array(w2066, w2083, w2082, w2081) -> (w2080:T35)
            n1364 = for {
              tunnel: w2102 -> [w2113]
              tunnel: w2080 -> [w2114] mode=indexing
              shift-right: [w2111] -> w2078
              shift-left: TRUE -> [w2112]
              shift-right: [w2110] -> w2076
              shift-left: _ -> [w2106]
              shift-right: [w2109] -> w2075
              shift-left: _ -> [w2105]
              shift-right: [w2108] -> w2074
              shift-left: _ -> [w2104]
              shift-right: [w2107] -> w2073
              shift-left: _ -> [w2103]
              n1365 = case shown="True" w2112 {
                selector: w2112 -> [w2119 _]
                tunnel: w2114 -> [_ w2128]
                tunnel: w2113 -> [_ w2126]
                tunnel: [w2119 w2124] -> w2111
                tunnel: [w2118 w2123] -> w2110
                tunnel: [w2117 w2122] -> w2109
                tunnel: [w2116 w2121] -> w2108
                tunnel: [w2115 w2120] -> w2107
                tunnel: w2106 -> [w2118 _]
                tunnel: w2105 -> [w2117 _]
                tunnel: w2104 -> [w2116 _]
                tunnel: w2103 -> [w2115 _]
                frame False {
                }
                frame True {
                  n1366 = Unbundle(w2128) -> (w2127:T34)
